vi "Start Capturing HTTP Method.vi"(8 "Error In":errorcluster, 9 "Start Capture":bool, 10 "Half capture time":u32=750) -> (0 "Error Out":errorcluster)   [LabVIEW 2014]
uses:
  FGV/Camer Control Variables.vi
  MicaSense RedEdge/Data And Commands/Capture Image/Capture Image.vi
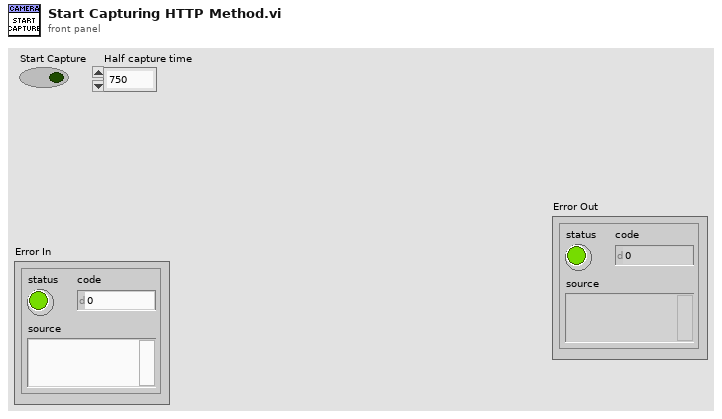
[diagram p1: front panel]
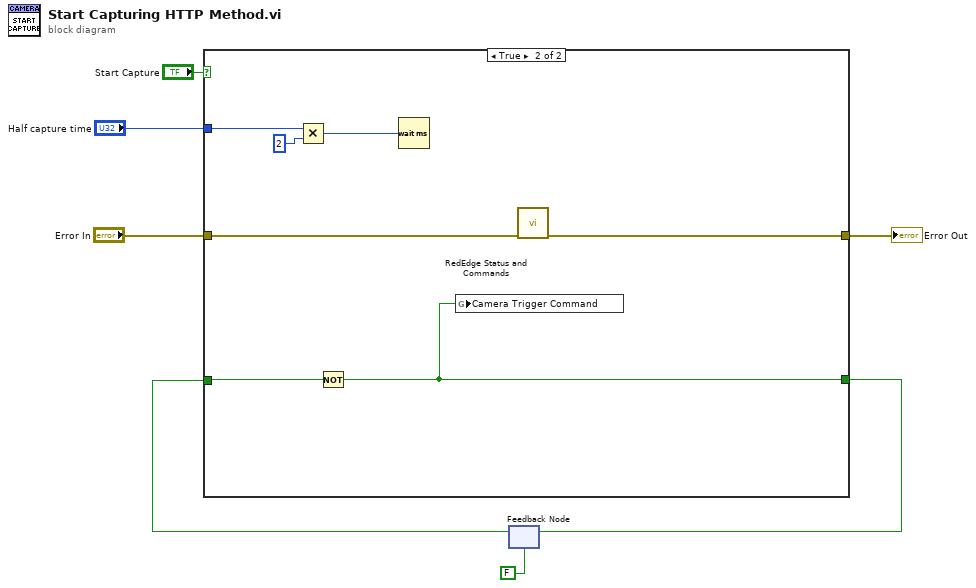
[diagram p0: block diagram]
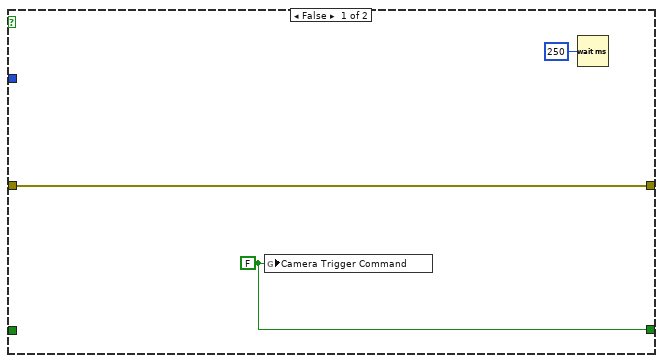
[diagram p2: hidden frame]
diagram:
  n1 = feedback #1(FALSE ("Camera Trigger Command")) -> (w2:bool)
  n2 = case shown="True" "Start Capture" {
    tunnel: "Error In" -> [w9 w14]
    tunnel: "Half capture time" -> [_ w17]
    tunnel: [w9 w13] -> w4
    tunnel: w2 -> [_ w12]
    tunnel: [w8 w11] -> w1
    frame False {
      w8 = FALSE ("Camera Trigger Command")
      n3 = global write "Camer Control Variables.vi" "Camera Trigger Command"(w8) -> ()
      n4 = Wait (ms)(milliseconds to wait=u32 250) -> ()  [unwired: 1 out]
    }
    frame True {
      n5 = Multiply(x=w17, y=u32 2) -> (x*y=w15:u32)
      n6 = Not(x=w12) -> (.not. x?=w11:bool)
      n7 = Wait (ms)(milliseconds to wait=w15) -> ()  [unwired: 1 out]
      n8 = global write "Camer Control Variables.vi" "Camera Trigger Command"(w11) -> ()
      n9 = call-poly "RedEdge Status and Commands.vi"("Error In"=w14) -> ("Error Out"=w13:errorcluster)  [unwired: 10 in]
    }
  }
  "Error Out" <- w4
  n10 = feedback-in #1(w1) -> ()
